vi "get devices with save variable.vi"(11 "List of devices":string[][](array[string])) -> (3 "array":string[][](array[string]))   [LabVIEW 2020]
uses:
  <userlib>/_OpenG.lib/array/array.llb/Filter 1D Array with Scalar (String)__ogtk.vi
panel:
  out "data":string[][](array[string])
  out "error out":errorcluster
  in  "error in (no error)":errorcluster
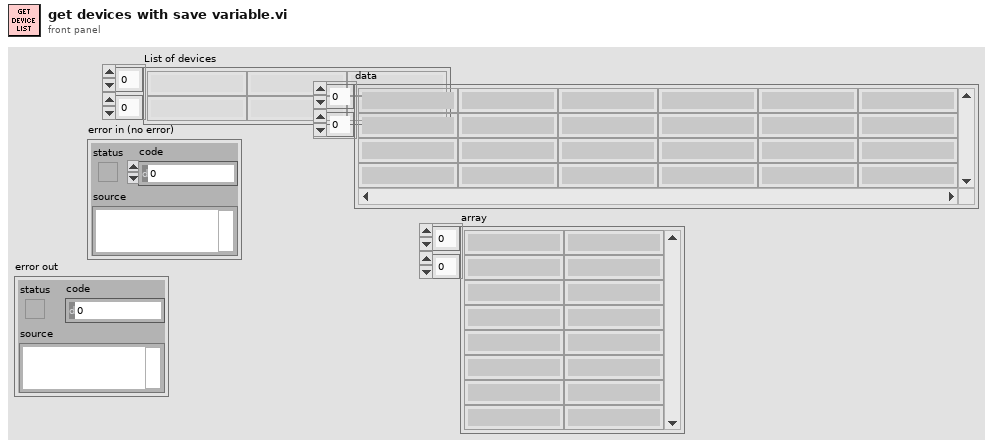
[diagram p1: front panel]
types:
  T1 = typedef "mysql_authentication.ctl" = cluster{"User":string, "Password":string, "Database":string}
  T2 = cluster{"Port":u16, "IP Address":string, "Authentication":T1}
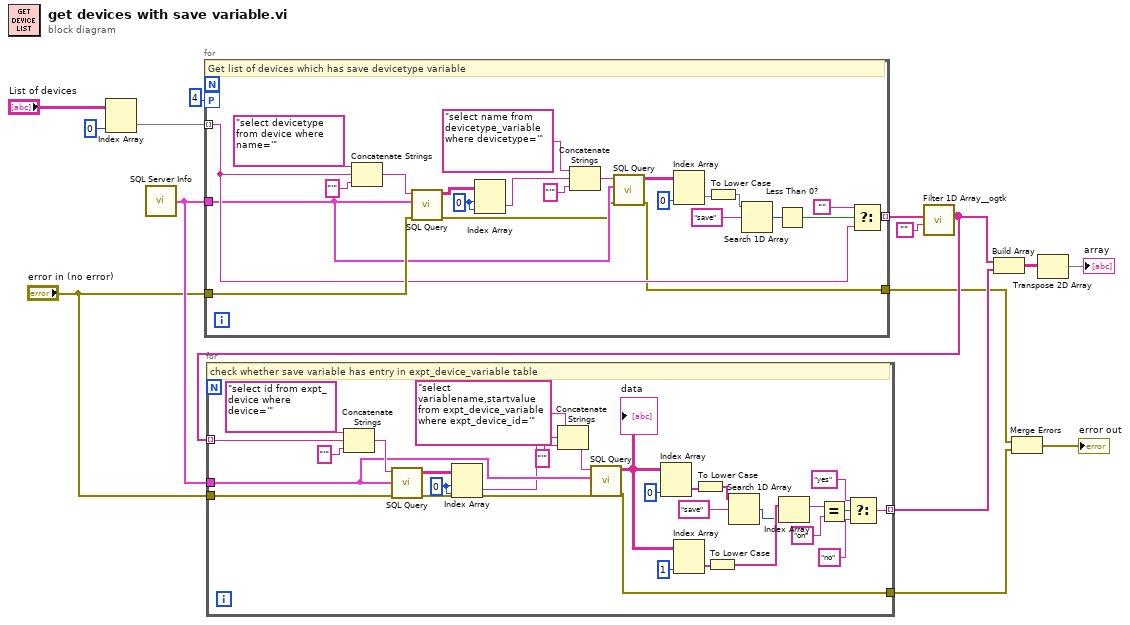
[diagram p0: block diagram]
diagram:
  n1 = Index Array(array="List of devices", index (col)=0 ("disabled index (col)")) -> (element=w7:string[])  [unwired: 1 in]
  n2 = call "SQL Server Info.vi"() -> ("SQL Server Info"=w8:T2)
  n3 = for {
    tunnel: w7 -> [w22] mode=indexing
    tunnel: "error in (no error)" -> [w35]
    tunnel: [w21] -> w13 mode=indexing
    workers-P: 4 -> [_]
    tunnel: w8 -> [w18]
    tunnel: [w16] -> w3
    w32 = 0 ("index (row)")
    # "Get list of devices which has save devicetype variable"
    n4 = Concatenate Strings("select devicetype from device where name='" ("Query"), w22, "'" ("Query")) -> (w36:string)
    n5 = call "SQL Query.vi"("error in (no error)"=w35, "SQL Server Info"=w18, "Query"=w36) -> ("error out"=w17:errorcluster, "data"=w33:string[][])  [unwired: 7 in]
    n6 = Index Array(array=w33, index (row)=w32, index (col)=w32) -> (element=w31:string)
    n7 = Concatenate Strings("select name from devicetype_variable where devicetype='" ("Query"), w31, "'" ("Query")) -> (w29:string)
    n8 = call "SQL Query.vi"("error in (no error)"=w17, "SQL Server Info"=w18, "Query"=w29) -> ("error out"=w16:errorcluster, "data"=w28:string[][])  [unwired: 7 in]
    n9 = Index Array(array=w28, index (col)=0 ("disabled index (col)")) -> (element=w25:string[])  [unwired: 1 in]
    n10 = To Lower Case(string=w25) -> (all lower case string=w24:string[])
    n11 = Search 1D Array(1D array=w24, element="save") -> (index of element=w23:i32)  [unwired: 1 in]
    n12 = Less Than 0?(x=w23) -> (x < 0?=w20:bool)
    n13 = Select(t="", s=w20, f=w22) -> (s? t:f=w21:string)
  }
  n14 = call-poly <userlib>:"Filter 1D Array__ogtk.vi"("items to filter"="", "array"=w13) -> ("filtered array"=w5:string[])  [unwired: 4 in, 1 out]
  n15 = for {
    tunnel: w8 -> [w60]
    tunnel: w5 -> [w65] mode=indexing
    tunnel: "error in (no error)" -> [w63]
    tunnel: [w54] -> w4 mode=indexing
    tunnel: [w39] -> w2
    w62 = 0 ("index (row)")
    # "check whether save variable has entry in expt_device_variable table"
    n16 = Concatenate Strings("select id from expt_device where device='" ("Query"), w65, "'" ("Query")) -> (w64:string)
    n17 = call "SQL Query.vi"("error in (no error)"=w63, "SQL Server Info"=w60, "Query"=w64) -> ("error out"=w59:errorcluster, "data"=w61:string[][])  [unwired: 7 in]
    n18 = Index Array(array=w61, index (row)=w62, index (col)=w62) -> (element=w52:string)
    n19 = Concatenate Strings("select variablename,startvalue from expt_device_variable where expt_device_id='" ("Query"), w52, "'" ("Query")) -> (w50:string)
    n20 = call "SQL Query.vi"("error in (no error)"=w59, "SQL Server Info"=w60, "Query"=w50) -> ("error out"=w39:errorcluster, "data"=w48:string[][])  [unwired: 7 in]
    "data" <- w48
    n21 = Index Array(array=w48, index (col)=0 ("disabled index (col)")) -> (element=w57:string[])  [unwired: 1 in]
    n22 = Index Array(array=w48, index (col)=1 ("disabled index (col)")) -> (element=w47:string[])  [unwired: 1 in]
    n23 = To Lower Case(string=w57) -> (all lower case string=w58:string[])
    n24 = To Lower Case(string=w47) -> (all lower case string=w46:string[])
    n25 = Search 1D Array(1D array=w58, element="save") -> (index of element=w40:i32)  [unwired: 1 in]
    n26 = Index Array(array=w46, index=w40) -> (element=w45:string)
    n27 = Equal?(x=w45, y="on" ("element")) -> (x = y?=w43:bool)
    n28 = Select(t="yes" ("element"), s=w43, f="no" ("element")) -> (s? t:f=w54:string)
  }
  n29 = Build Array(w5, w4) -> (w11:string[][])
  n30 = Merge Errors(w3, w2) -> (→"error out":errorcluster)
  n31 = Transpose 2D Array(2D array=w11) -> (transposed array=→"array":string[][])
